vi "Unpacking data.vi"(8 "error in (no error)":errorcluster, 11 "data in":string) -> (0 "error out":errorcluster, 1 "trimmed string":string, 2 "Numeric":dbl, 3 "Cluster":T1)   [LabVIEW 2022 SP3]
uses:
  <vilib>/Utility/error.llb/Trim Whitespace One-Sided.vi
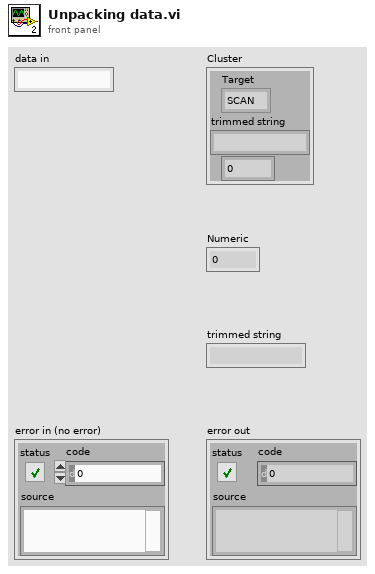
[diagram p1: front panel]
types:
  T1 = cluster{"Target":enum16{"SCAN", "TDC", "CAM", "POW", "LOG", "ANLYS", "VOLT", "MOTOR", "DELAY", "LASER"}, "trimmed string":string, dbl}
  T2 = enum16{"SCAN", "TDC", "CAM", "POW", "LOG", "ANLYS", "VOLT", "MOTOR", "DELAY", "LASER"}
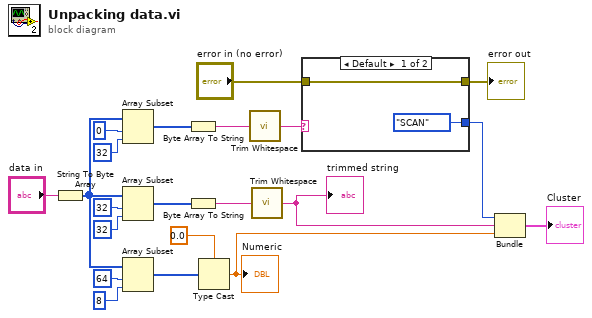
[diagram p0: block diagram]
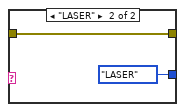
[diagram p2: hidden frame]
diagram:
  n1 = String To Byte Array(string="data in") -> (unsigned byte array=w9:u8[])
  n2 = Array Subset(array=w9, index=0, length=32) -> (w8:u8[])
  n3 = Array Subset(array=w9, index=32, length=32) -> (w7:u8[])
  n4 = Array Subset(array=w9, index=64, length=8) -> (w6:u8[])
  n5 = Byte Array To String(unsigned byte array=w8) -> (string=w4:string)
  n6 = Byte Array To String(unsigned byte array=w7) -> (string=w5:string)
  n7 = Type Cast(type=0.0, x=w6) -> (*(type *) &x=w21:dbl)
  "Numeric" <- w21
  n8 = call <vilib>:"Trim Whitespace.vi"("string"=w4) -> ("trimmed string"=w3:string)  [unwired: 1 in]
  n9 = call <vilib>:"Trim Whitespace.vi"("string"=w5) -> ("trimmed string"=w20:string)  [unwired: 1 in]
  "trimmed string" <- w20
  n10 = case shown="Default" w3 {
    tunnel: [T2."SCAN" ("Target") T2."LASER" ("Target")] -> w2
    tunnel: "error in (no error)" -> [w22 w24]
    tunnel: [w22 w24] -> w18
    frame Default {
    }
    frame "LASER" {
    }
  }
  "error out" <- w18
  n11 = Bundle("Target"=w2, "trimmed string"=w20, w21) -> (→"Cluster":T1)  [unwired: 1 in]
